vi "PH_Calorimeter_USB.set i Attr.vi"(0 "i ref in":refnum<vi>, 5 "error in (no error)":errorcluster) -> (14 "i ref out":refnum<vi>, 17 "i Attributes":T1={"GUI Refs"={"Delete"=refnum, "Start"=refnum, "Energy"=refnum, "Calorimeter"=refnum, "Trigger"=refnum, "Calo Calibration"=refnum, "Time Base"=refnum, "Device"=refnum, "Graph Raw Data"=refnum, "Graph Result"=refnum}, "DAQ Instance"="N/A", "Data"=[], "Controller Instance"="N/A", "Energy [J]"=0.0, "Calorimeter"={"Channel"="Dev1/ai1", "Min Value [V]"=-1.0, "Max Value  [V]"=1.0}, "Trigger"={"Channel"="", "Min Value [V]"=-10.0, "Max Value  [V]"=10.0, "Level [V]"=1.0, "Wait Time [s]"=60.0, "Length [Samples]"=10}, "Time Base"={"Samples per Channel"=28000, "Rate [Hz]"=100}, "Calo Calibration"={"T 1/e [s]"=220.0, "Sensitivity  [Vs/J]"=0.0592}, "Serial Number"="N/A"} {"Calo Calibration"."Sensitivity  [Vs/J]" format="%.4f"; "Trigger"."Level [V]" format="%0.2f"; "Trigger"."Max Value  [V]" format="%0.2f"; "Trigger"."Min Value [V]" format="%0.2f"; "Calorimeter"."Max Value  [V]" format="%0.2f"; "Calorimeter"."Min Value [V]" format="%0.2f"}, 19 "error out":errorcluster)   [LabVIEW 2014, in "PH_Calorimeter_USB.lvlib"]
doc: "This VI gets information from the data base and input, sets the attributes and the related GUI elements."
uses:
  PH_Calorimeter_USB.lvlib
  PH_Calorimeter_USB.i attribute.ctl
  PH_Calorimeter_USB.Calorimeter Settings.ctl
  PH_Calorimeter_USB.Trigger Settings.ctl
  PH_Calorimeter_USB.Time Base Settings.ctl
  PH_Calorimeter_USB.Calorimeter Calibration Settings.ctl
  CSCore/CSSystem/CSSystemLib/CSSystemLib.lvlib
  PH_Common/PH_Common.lvlib
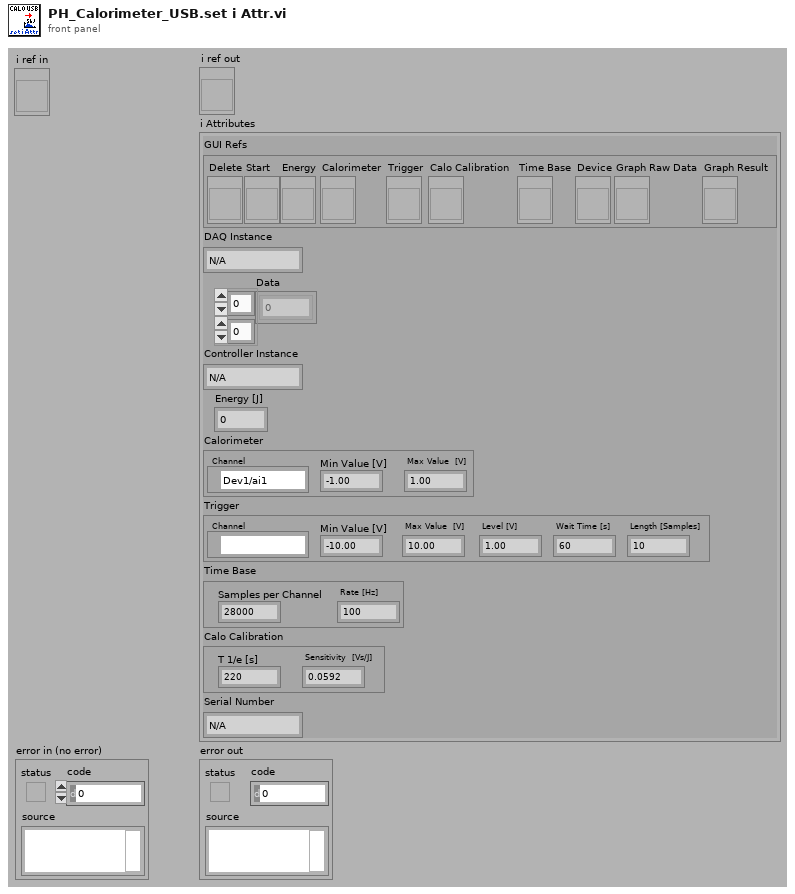
[diagram p1: front panel]
types:
  T1 = typedef "PH_Calorimeter_USB.lvlib/PH_Calorimeter_USB.i attribute.ctl" = cluster{"GUI Refs":cluster{"Delete":refnum<vi>, "Start":refnum<vi>, "Energy":refnum<vi>, "Calorimeter":refnum<vi>, "Trigger":refnum<vi>, "Calo Calibration":refnum<vi>, "Time Base":refnum<vi>, "Device":refnum<vi>, "Graph Raw Data":refnum<vi>, "Graph Result":refnum<vi>}, "DAQ Instance":string, "Data":dbl[][], "Controller Instance":string, "Energy [J]":dbl, "Calorimeter":T2, "Trigger":T3, "Time Base":T4, "Calo Calibration":T5, "Serial Number":string}
  T2 = typedef "PH_Calorimeter_USB.lvlib/PH_Calorimeter_USB.Calorimeter Settings.ctl" = cluster{"Channel":tag, "Min Value [V]":dbl, "Max Value  [V]":dbl}
  T3 = typedef "PH_Calorimeter_USB.lvlib/PH_Calorimeter_USB.Trigger Settings.ctl" = cluster{"Channel":tag, "Min Value [V]":dbl, "Max Value  [V]":dbl, "Level [V]":dbl, "Wait Time [s]":dbl, "Length [Samples]":i32}
  T4 = typedef "PH_Calorimeter_USB.lvlib/PH_Calorimeter_USB.Time Base Settings.ctl" = cluster{"Samples per Channel":i32, "Rate [Hz]":i32}
  T5 = typedef "PH_Calorimeter_USB.lvlib/PH_Calorimeter_USB.Calorimeter Calibration Settings.ctl" = cluster{"T 1/e [s]":dbl, "Sensitivity  [Vs/J]":dbl}
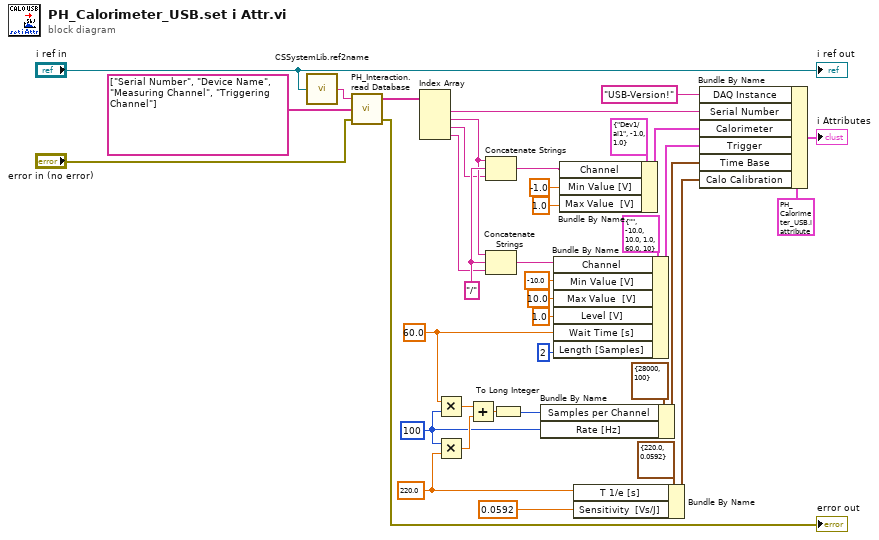
[diagram p0: block diagram]
diagram:
  w13 = "/" ("string")
  w16 = 220.0 ("T 1/e [s]")
  w18 = 100 ("Rate [Hz]")
  w17 = 60.0 ("Wait Time [s]")
  n1 = call "CSSystemLib.ref2name.vi"("obj refnum"="i ref in") -> ("name"=w8:string)
  n2 = call "PH_Interaction.read Database.vi"("error in (no error)"="error in (no error)", "Strings to search for"=string[] ["Serial Number", "Device Name", "Measuring Channel", "Triggering Channel"], "DB Entry to read"=w8) -> ("error out"=→"error out":errorcluster, "Values"=w5:string[])  [unwired: 1 in]
  n3 = Index Array(array=w5) -> (element #1=w37:string, element #2=w4:string, element #3=w3:string, element #4=w2:string)  [unwired: 4 in]
  n4 = Multiply(x=w17, y=w18) -> (x*y=w22:dbl)
  n5 = Multiply(x=w18, y=w16) -> (x*y=w21:dbl)
  n6 = Add(x=w22, y=w21) -> (x+y=w20:dbl)
  n7 = Concatenate Strings(w4, w13, w3) -> (w12:string)
  n8 = Concatenate Strings(w4, w13, w2) -> (w11:string)
  n9 = To Long Integer(number=w20) -> (32bit integer=w19:i32)
  n10 = Bundle By Name(cluster=T4 {"Samples per Channel"=28000, "Rate [Hz]"=100} ("Time Base"), "Samples per Channel"=w19, "Rate [Hz]"=w18) -> (w26:T4)
  n11 = Bundle By Name(cluster=T3 {"Channel"="", "Min Value [V]"=-10.0, "Max Value  [V]"=10.0, "Level [V]"=1.0, "Wait Time [s]"=60.0, "Length [Samples]"=10} ("Trigger"), "Channel"=w11, "Min Value [V]"=-10.0, "Max Value  [V]"=10.0, "Level [V]"=1.0, "Wait Time [s]"=w17, "Length [Samples]"=2) -> (w28:T3)
  n12 = Bundle By Name(cluster=T2 {"Channel"="Dev1/ai1", "Min Value [V]"=-1.0, "Max Value  [V]"=1.0} ("Calorimeter"), "Channel"=w12, "Min Value [V]"=-1.0, "Max Value  [V]"=1.0) -> (w15:T2)
  n13 = Bundle By Name(cluster=T5 {"T 1/e [s]"=220.0, "Sensitivity  [Vs/J]"=0.0592} ("Calo Calibration"), "T 1/e [s]"=w16, "Sensitivity  [Vs/J]"=0.0592) -> (w24:T5)
  n14 = Bundle By Name(cluster=T1 {"GUI Refs"={"Delete"=refnum, "Start"=refnum, "Energy"=refnum, "Calorimeter"=refnum, "Trigger"=refnum, "Calo Calibration"=refnum, "Time Base"=refnum, "Device"=refnum, "Graph Raw Data"=refnum, "Graph Result"=refnum}, "DAQ Instance"="N/A", "Data"=[], "Controller Instance"="N/A", "Energy [J]"=0.0, "Calorimeter"={"Channel"="Dev1/ai1", "Min Value [V]"=-1.0, "Max Value  [V]"=1.0}, "Trigger"={"Channel"="", "Min Value [V]"=-10.0, "Max Value  [V]"=10.0, "Level [V]"=1.0, "Wait Time [s]"=60.0, "Length [Samples]"=10}, "Time Base"={"Samples per Channel"=28000, "Rate [Hz]"=-1}, "Calo Calibration"={"T 1/e [s]"=220.0, "Sensitivity  [Vs/J]"=-10.0}, "Serial Number"="N/A"} ("i attribute"), "DAQ Instance"="USB-Version!", "Serial Number"=w37, "Calorimeter"=w15, "Trigger"=w28, "Time Base"=w26, "Calo Calibration"=w24) -> (→"i Attributes":T1)
  "i ref out" <- "i ref in"
